vi "OdometerWrite.vi"(8 "error in (no error)":errorcluster caption="Fehler (Eingang, kein Fehler)", 10 "Numerisch":dbl, 11 "configuration file path":path caption="Pfad der Konfigurationsdatei") -> (0 "error out":errorcluster caption="Fehler (Ausgang)", 3 "file path":path caption="Dateipfad")   [LabVIEW 2013]
uses:
  <vilib>/Utility/config.llb/Write Key (Double).vi
  <vilib>/Utility/config.llb/NI_LVConfig.lvlib
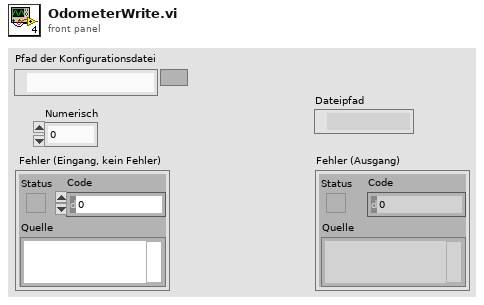
[diagram p1: front panel]
types:
  T1 = typedef "NI_LVConfig.lvlib/Config Data RefNum.ctl" = refnum<k1>
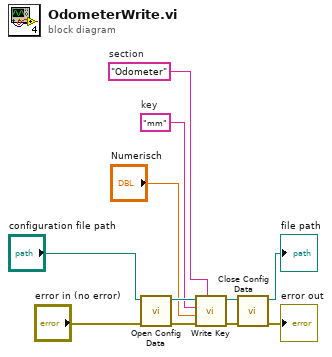
[diagram p0: block diagram]
diagram:
  w6 = "mm"  # key
  w7 = "Odometer"  # section
  n1 = call <vilib>:"Open Config Data.vi"("error in (no error)"="error in (no error)", "configuration file path"="configuration file path") -> ("error out"=w10:errorcluster, "refnum"=w11:T1)  [unwired: 7 in, 1 out]
  n2 = call-poly <vilib>:"Write Key.vi"("section"=w7, "error in (no error)"=w10, "value"="Numerisch", "key"=w6, "refnum"=w11) -> ("error out"=w9:errorcluster, "refnum out"=w8:T1)  [unwired: 4 in, 1 out]
  n3 = call <vilib>:"Close Config Data.vi"("error in (no error)"=w9, "refnum"=w8) -> ("error out"=→"error out":errorcluster, "file path"=→"file path":path)  [unwired: 8 in]
